vi "set z_intensity tupels.vi"(8 "error in (no error)":errorcluster, 10 "z/intensity tupesl IN":u32[](array[numeric]), 11 "TrajectoryAK101022Resonance in":refnum<class "TrajectoryAK101022Resonance.lvclass">) -> (0 "error out":errorcluster, 3 "TrajectoryAK101022Resonance out":refnum<class "TrajectoryAK101022Resonance.lvclass">)   [LabVIEW 2010, in "TrajectoryAK101022Resonance.lvclass"]
uses:
  TrajectoryAK101022Resonance.lvclass
  TrajectoryAK101022Resonance.lvclass/TrajectoryAK101022Resonance.ctl
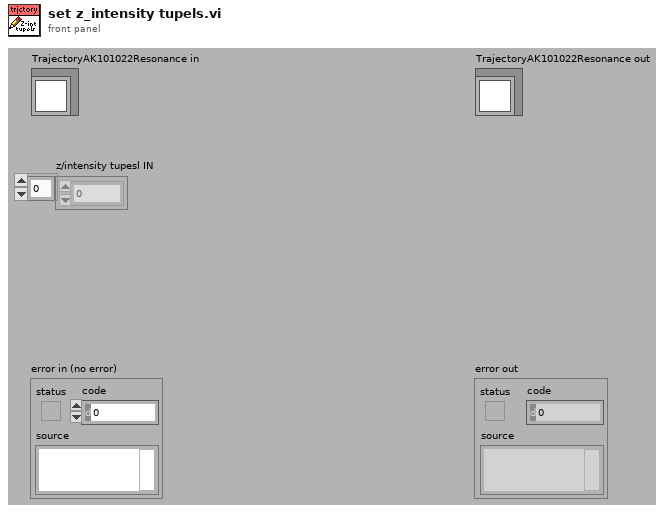
[diagram p1: front panel]
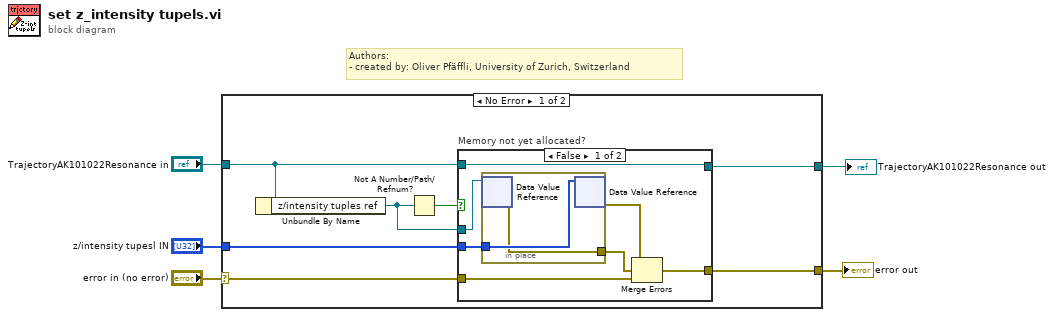
[diagram p0: block diagram]
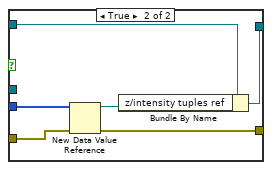
[diagram p2: hidden frame]
diagram:
  # "Authors: \n- created by: Oliver Pfäffli, University of Zurich, Switzerland"
  n1 = case shown="No Error" "error in (no error)" {
    selector: "error in (no error)" -> [w7 w29]
    tunnel: [w6 w29] -> w4
    tunnel: [w9 w28] -> w2
    tunnel: "TrajectoryAK101022Resonance in" -> [w10 w28]
    tunnel: "z/intensity tupesl IN" -> [w11 _]
    frame No Error {
      n2 = Unbundle By Name(w10) -> ("z/intensity tuples ref"=w8:refnum<data-value>)
      n3 = Not A Number/Path/Refnum?(number/path/refnum=w8) -> (NaN/Path/Refnum?=w12:bool)
      n4 = case "Memory not yet allocated?" shown="False" w12 {
        tunnel: w11 -> [w19 w24]
        tunnel: w10 -> [w18 w26]
        tunnel: [w18 w25] -> w9
        tunnel: w8 -> [w17 _]
        tunnel: w7 -> [w14 w23]
        tunnel: [w13 w22] -> w6
        frame False {
          n5 = in-place {
            in-place-border: w19 -> [w21]
            in-place-border: [w20] -> w16
            n6 = in-place-dvr #1(w17) -> (w20:errorcluster)  [unwired: 1 out]
            n7 = in-place-dvr #1(w21) -> (w15:errorcluster)  [unwired: 1 out]
          }
          n8 = Merge Errors(w15, w16, w14) -> (w13:errorcluster)
        }
        frame True {
          n9 = New Data Value Reference(data value=w24, error in=w23) -> (data value reference=w27:refnum<data-value>, error out=w22:errorcluster)
          n10 = Bundle By Name(cluster=w26, "z/intensity tuples ref"=w27) -> (w25:refnum<class "TrajectoryAK101022Resonance.lvclass">)
        }
      }
    }
    frame Error {
    }
  }
  "error out" <- w4
  "TrajectoryAK101022Resonance out" <- w2
